vi "HEWH RLT PRAT.vi"() -> ()   [LabVIEW 2016] (continued)
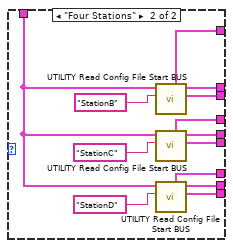
[diagram p3: hidden frame]
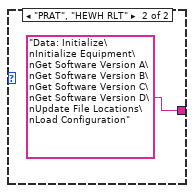
[diagram p4: hidden frame]
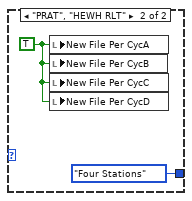
[diagram p5: hidden frame]
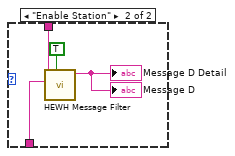
[diagram p6: hidden frame]
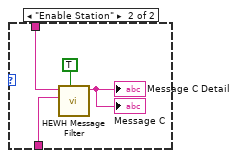
[diagram p7: hidden frame]
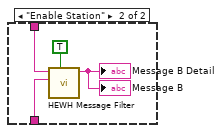
[diagram p8: hidden frame]
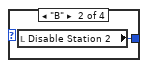
[diagram p10: hidden frame]
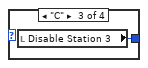
[diagram p11: hidden frame]
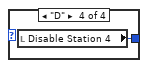
[diagram p12: hidden frame]
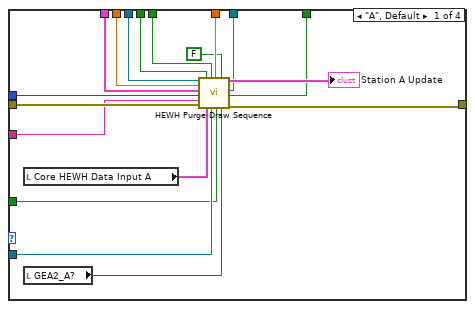
[diagram p14: hidden frame]
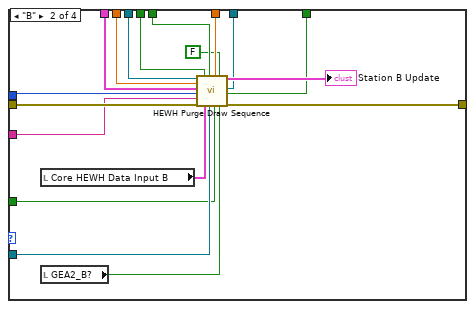
[diagram p15: hidden frame]
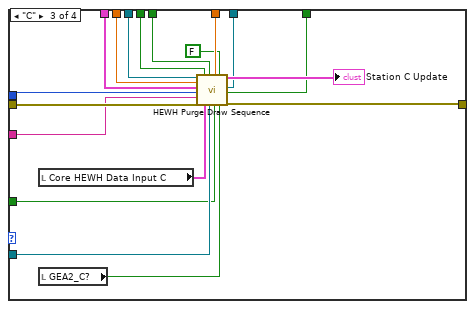
[diagram p16: hidden frame]
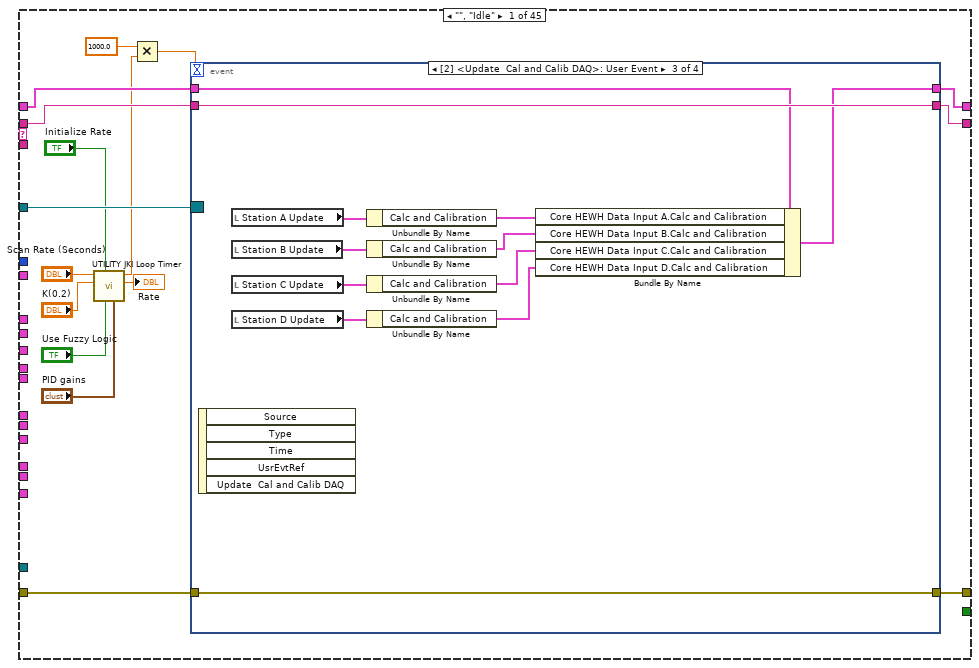
[diagram p18: hidden frame]
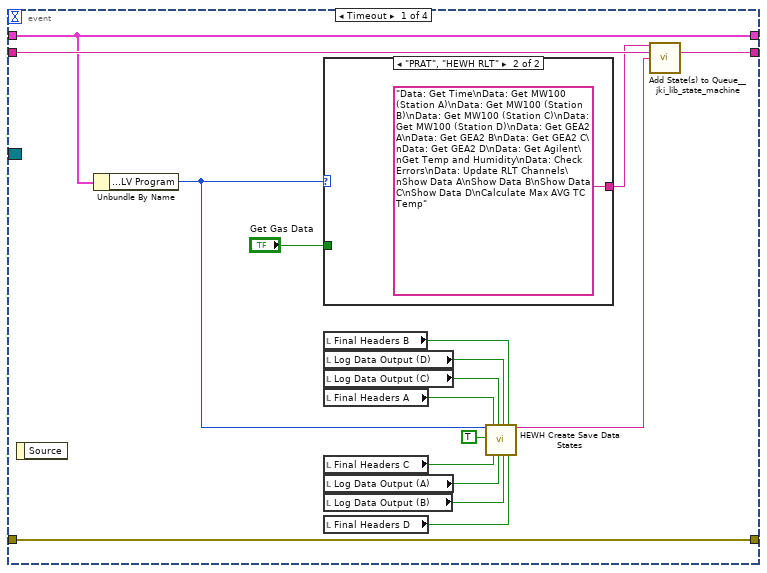
[diagram p19: hidden frame]
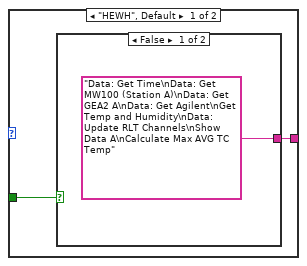
[diagram p20: hidden frame]
        n1683 = Bundle By Name(cluster=w3884, "Alarms.T-Out Over A"=w3918, "Alarms.T-Out Over B"=w3919, "Alarms.T-Out Over C"=w3920, "Alarms.T-Out Over D"=w3921) -> (w3882:T86)
        n1684 = Compound Arithmetic op=OR(w3908, w3909, w3910, w3911) -> (w3912:bool)
        n1685 = case shown="True" w3912 {
          tunnel: ["" "Save Error Data"] -> w3907
          frame False {
          }
          frame True {
          }
        }
        n1686 = call <vilib>:"Add State(s) to Queue__jki_lib_state_machine.vi"("State(s) in Front (\"\")"=w3907, "State(s) in (\"\")"=w3883) -> ("States Out"=w3881:string)  [unwired: 13 in]
      }
      frame "Save Error Data" {
        # "If \"EEV or T-OUT over limit\" error occurs, log to C:\\Data\\Errors.csv file"
        n1687 = local read "Alarm B"() -> (w3931:bool)
        n1688 = local read "Alarm A"() -> (w3930:bool)
        n1689 = local read "Alarm C"() -> (w3932:bool)
        n1690 = local read "Alarm D"() -> (w3933:bool)
        n1691 = case shown="True" w3933 {
          frame False {
          }
          frame True {
            n1692 = local read "EEV Over D"() -> (w3935:bool)
            n1693 = local read "T-OUT Over D"() -> (w3934:bool)
            n1694 = call "HEWH Errors Save to File.vi"("EEV Over A"=w3935, "T-OUT Over A"=w3934) -> ()  [unwired: 8 in, 1 out]
          }
        }
        n1695 = case shown="True" w3930 {
          frame False {
          }
          frame True {
            n1696 = local read "EEV Over A"() -> (w3941:bool)
            n1697 = local read "T-OUT Over A"() -> (w3940:bool)
            n1698 = call "HEWH Errors Save to File.vi"("EEV Over A"=w3941, "T-OUT Over A"=w3940) -> ()  [unwired: 8 in, 1 out]
          }
        }
        n1699 = case shown="True" w3931 {
          frame False {
          }
          frame True {
            n1700 = local read "EEV Over B"() -> (w3939:bool)
            n1701 = local read "T-OUT Over B"() -> (w3938:bool)
            n1702 = call "HEWH Errors Save to File.vi"("EEV Over A"=w3939, "T-OUT Over A"=w3938) -> ()  [unwired: 8 in, 1 out]
          }
        }
        n1703 = case shown="True" w3932 {
          frame False {
          }
          frame True {
            n1704 = local read "EEV Over C"() -> (w3937:bool)
            n1705 = local read "T-OUT Over C"() -> (w3936:bool)
            n1706 = call "HEWH Errors Save to File.vi"("EEV Over A"=w3937, "T-OUT Over A"=w3936) -> ()  [unwired: 8 in, 1 out]
          }
        }
        n1707 = call <vilib>:"Add State(s) to Queue__jki_lib_state_machine.vi"("State(s) in (\"\")"=w3928) -> ("States Out"=w3926:string)  [unwired: 14 in]
      }
      frame "Clear Errors" {
        w3946 = FALSE
        n1708 = Bundle By Name(cluster=w3943, "Alarms.EEV Over A"=w3946, "Alarms.EEV Over B"=w3946, "Alarms.EEV Over C"=w3946, "Alarms.EEV Over D"=w3946, "Alarms.T-Out Over A"=w3946, "Alarms.T-Out Over B"=w3946, "Alarms.T-Out Over C"=w3946, "Alarms.T-Out Over D"=w3946) -> (w3942:T86)
      }
    }
  }
  n1709 = call "GEA2 Stop.vi"("GEA2 Reference Out"=w42, "Error In"=w120) -> ("Error Out"=w91:errorcluster)  [unwired: 13 in]
  n1710 = call "GEA2 Stop.vi"("GEA2 Reference Out"=w43, "Error In"=w120) -> ("Error Out"=w90:errorcluster)  [unwired: 13 in]
  n1711 = call "GEA2 Stop.vi"("GEA2 Reference Out"=w44, "Error In"=w120) -> ("Error Out"=w89:errorcluster)  [unwired: 13 in]
  n1712 = call "GEA2 Stop.vi"("GEA2 Reference Out"=w45, "Error In"=w120) -> ("Error Out"=w88:errorcluster)  [unwired: 13 in]
  n1713 = Merge Errors(w91, w90, w89, w88) -> (w87:errorcluster)
  n1714 = Unregister For Events(event registration refnum=w86, error in=w87) -> ()  [unwired: 1 out]
  n1715 = property on="Finish" class="Bool (strict)"("Val(Sgnl)"=w128) -> ()  [unwired: 2 in, 2 out]
  n1716 = Release Queue(queue=w118, error in (no error)=w117) -> (error out=→"Error Out":errorcluster)  [unwired: 1 in, 2 out]
  n1717 = disable-structure shown="Disabled" {
    frame Disabled {
      n1718 = local read "Yokogawa WT210"() -> (w3947:refnum<visa-resource-name>)
      n1719 = local read "MW100"() -> (w3948:refnum<visa-resource-name>)
      n1720 = call "HEWH Runtime Wh Reset.vi"("Yokogawa WT210"=w3947, "MW100"=w3948) -> ()  [unwired: 9 in, 1 out]
    }
    frame Enabled {
    }
  }
